vi "TDTRX6-Read Data.vi"(1 "Action":T1=enum."Read", 7 "Pts Per Read":i32, 11 "error in (no error)":errorcluster, 12 "AI Channels":i32[](array[numeric])=[1, 2]) -> (10 "AI Waveforms":dbl[][](array[numeric]), 15 "error out":errorcluster)   [LabVIEW 2015]
uses:
  TDT-Signal Bank Action.ctl
  TDT-Globals.vi
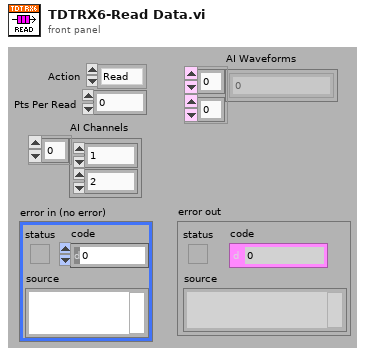
[diagram p1: front panel]
types:
  T1 = typedef "TDT-Signal Bank Action.ctl" = enum16{"Init", "Write", "Read", "Rewrite", "Reset", "Recycle", "Ramp up", "Ramp down", "Zero"}
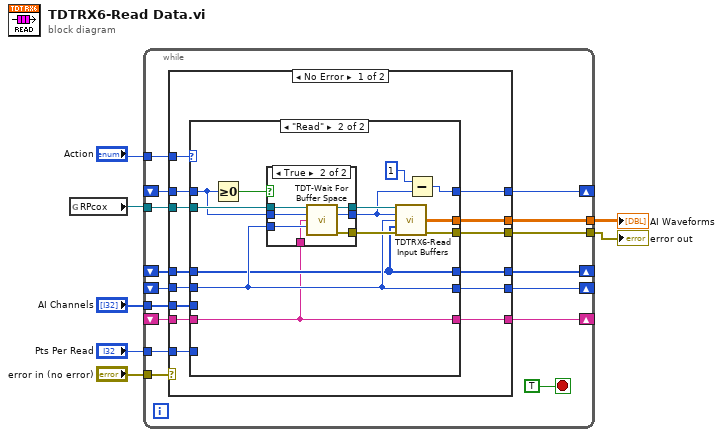
[diagram p0: block diagram]
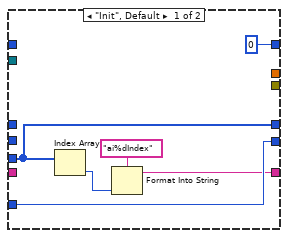
[diagram p2: hidden frame]
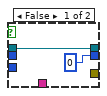
[diagram p3: hidden frame]
diagram:
  n1 = global read "TDT-Globals.vi" "RPcox"() -> (w5:refnum<k7>)
  n2 = while {
    tunnel: [w23] -> w6
    tunnel: "error in (no error)" -> [w22]
    tunnel: w5 -> [w21]
    tunnel: "Action" -> [w20]
    shift-right: [w18] -> _
    shift-left: _ -> [w17]
    tunnel: "Pts Per Read" -> [w16]
    shift-right: [w15] -> _
    shift-left: _ -> [w14]
    tunnel: [w13] -> w2
    tunnel: "AI Channels" -> [w12]
    shift-right: [w11] -> _
    shift-left: _ -> [w10]
    shift-right: [w9] -> _
    shift-left: _ -> [w8]
    stop <- TRUE stop-if-true
    n3 = case shown="No Error" w22 {
      selector: w22 -> [_ w70]
      tunnel: [w33 w70] -> w23
      tunnel: w21 -> [w34 _]
      tunnel: w20 -> [w37 _]
      tunnel: [w36 w69] -> w18
      tunnel: w17 -> [w35 w69]
      tunnel: w16 -> [w32 _]
      tunnel: [w31 w68] -> w15
      tunnel: w14 -> [w30 w68]
      tunnel: [w29 _] -> w13
      tunnel: w12 -> [w28 _]
      tunnel: [w27 w67] -> w11
      tunnel: w10 -> [w26 w67]
      tunnel: [w25 w66] -> w9
      tunnel: w8 -> [w24 w66]
      frame No Error {
        n4 = case shown="\"Read\"" w37 {
          tunnel: [0 w56] -> w36
          tunnel: w35 -> [_ w49]
          tunnel: w34 -> [_ w53]
          tunnel: [_ w51] -> w33
          tunnel: w32 -> [w42 _]
          tunnel: [w42 w46] -> w31
          tunnel: w30 -> [_ w46]
          tunnel: [_ w47] -> w29
          tunnel: w28 -> [w41 _]
          tunnel: [w41 w45] -> w27
          tunnel: w26 -> [_ w45]
          tunnel: [w38 w44] -> w25
          tunnel: w24 -> [_ w44]
          frame "Init", Default {
            n5 = Index Array(array=w41) -> (element=w39:i32)  [unwired: 1 in]
            n6 = Format Into String(format string="ai%dIndex", w39) -> (resulting string=w38:string)  [unwired: 2 in, 1 out]
          }
          frame "Read" {
            n7 = Greater Or Equal To 0?(x=w49) -> (x >= 0?=w48:bool)
            n8 = case shown="True" w48 {
              tunnel: [_ w65] -> w54
              tunnel: w53 -> [w58 w64]
              tunnel: [w58 w63] -> w52
              tunnel: w49 -> [_ w62]
              tunnel: [0 ("Next Buffer Out") w61] -> w50
              tunnel: w46 -> [_ w60]
              tunnel: w44 -> [_ w59]
              frame False {
              }
              frame True {
                n9 = call "TDT-Wait For Buffer Space.vi"("RPcox"=w64, "Next Buffer"=w62, "Tag"=w59, "Buffer Length"=w60) -> ("RPcox Out"=w63:refnum<k7>, "Next Buffer thru"=w61:i32, "error out"=w65:errorcluster)  [unwired: 9 in]
              }
            }
            n10 = call "TDTRX6-Read Input Buffers.vi"("RPcox"=w52, "Next Buffer"=w50, "Pts Per Read"=w46, "AI Channels"=w45, "error in (no error)"=w54) -> ("Input array"=w47:dbl[][], "error out"=w51:errorcluster)  [unwired: 9 in]
            n11 = Subtract(x=1, y=w50) -> (x-y=w56:i32)
          }
        }
      }
      frame Error {
      }
    }
  }
  "error out" <- w6
  "AI Waveforms" <- w2
